vi "CRYGet Scale in Curves.vi"(11 "Graph VI Ref":refnum<vi>) -> (0 "Y min":dbl, 1 "Y max":dbl, 2 "X min":dbl, 3 "X max":dbl)   [LabVIEW 2013]
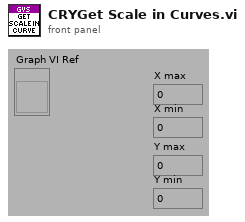
[diagram p1: front panel]
types:
  T1 = typedef "CRYData Cluster.ctl" = cluster{"Name":string, "Curve":cluster{"x":dbl, "y":dbl, "z":dbl}[], "X data":u16, "Y data":u16, "Z data":u16, "X axis":u16, "Y axis":u16, "Z axis":u16, "X unit":string, "Y unit":string, "Z unit":string, "X dB ref":dbl, "Y dB ref":dbl, "Z dB ref":dbl, "single val":bool, "protected":bool, "display X":bool, "display Y":bool, "display Z":bool, "Test Info":string, "Step No.":i32, "Plot Settings":cluster{"Color":u32, "Interpolation":u8, "Point Style":u8, "Line Style":u8, "Point Color":u32, "Line Width":u8, "Bar Plot Style":u8, "Fill To":i16}, "AutoProtect":bool}
  T2 = typedef "CRYWaveform Cluster.ctl" = cluster{"Waveform":cluster{"X0":dbl, "dX":dbl, "Y":sgl[]}, "X data":u16, "Y data":u16, "Y axis":u16, "X unit":string, "Y unit":string, "Y dB ref":dbl, "display Y":bool, "display X":bool, "Overload?":bool, "Test Info":string, "Step No.":i32, "Name":string, "protected":bool, "Sqc history":string[], "Signal Channel ID":i32, "Plot Settings":cluster{"Color":u32, "Interpolation":u8, "Point Style":u8, "Line Style":u8, "Point Color":u32, "Line Width":u8, "Bar Plot Style":u8, "Fill To":i16}, "AutoProtect":bool}
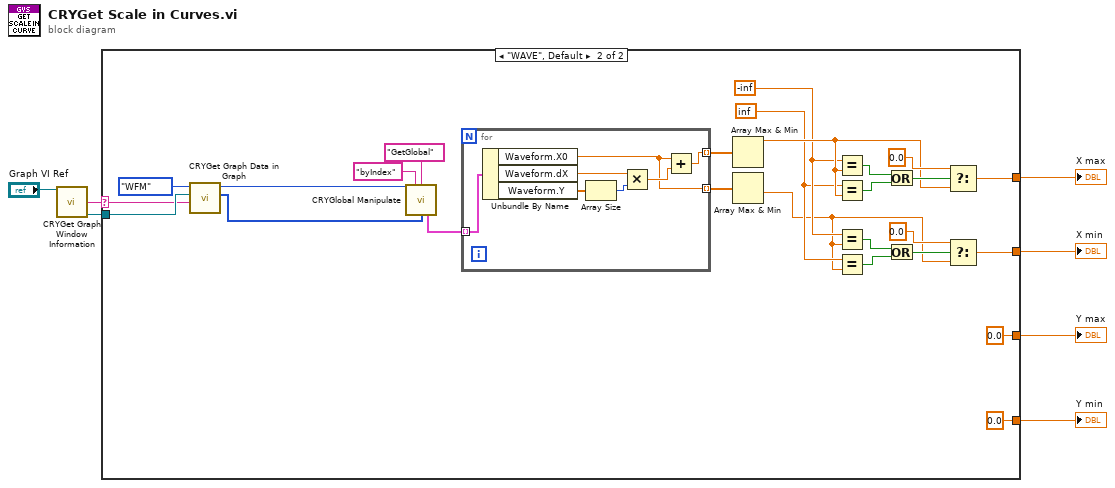
[diagram p0: block diagram]
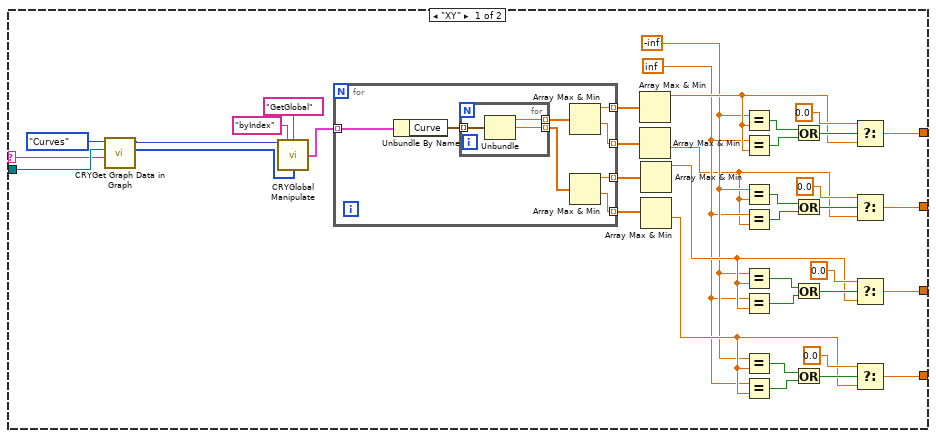
[diagram p2: hidden frame]
diagram:
  n1 = call "CRYGet Graph Window Information.vi"("pGraph VI In"="Graph VI Ref") -> ("Graph Type Out"=w2:string, "Legend Ref Out"=w1:refnum<vi>)  [unwired: 4 in, 9 out]
  n2 = case shown="\"WAVE\", Default" w2 {
    selector: w2 -> [w13 w64]
    tunnel: [w36 w75] -> w7
    tunnel: [w31 w70] -> w6
    tunnel: [w26 0.0 ("max value")] -> w5
    tunnel: [w21 0.0 ("max value")] -> w4
    tunnel: w1 -> [w14 w65]
    frame "XY" {
      w18 = -inf
      w17 = inf
      n3 = call "CRYGet Graph Data in Graph.vi"("Graph Type"=w13, "Legend Refnum"=w14, "Type In"=enum16{"Curves", "Values", "Results", "WFM"}."Curves") -> ("Rows"=w8:i32[], "Type Out"=w9:enum16{"Curves", "Values", "Results", "WFM"})  [unwired: 4 in, 3 out]
      n4 = call "CRYGlobal Manipulate.vi"("Type"=w9, "sOption"="byIndex", "sAction"="GetGlobal", "nData"=w8) -> ("Curves Out"=w11:T1[])  [unwired: 5 in, 6 out]
      n5 = for {
        tunnel: [w50] -> w42 mode=indexing
        tunnel: [w49] -> w43 mode=indexing
        tunnel: [w48] -> w44 mode=indexing
        tunnel: [w47] -> w45 mode=indexing
        tunnel: w11 -> [w46] mode=indexing
        n6 = Unbundle By Name(w46) -> ("Curve"=w53:cluster{"x":dbl, "y":dbl, "z":dbl}[])
        n7 = for {
          tunnel: w53 -> [w56] mode=indexing
          tunnel: [w55] -> w52 mode=indexing
          tunnel: [w54] -> w51 mode=indexing
          n8 = Unbundle(w56) -> ("x"=w55:dbl, "y"=w54:dbl)  [unwired: 1 out]
        }
        n9 = Array Max & Min(array=w52) -> (max value=w50:dbl, min value=w48:dbl)  [unwired: 2 out]
        n10 = Array Max & Min(array=w51) -> (max value=w49:dbl, min value=w47:dbl)  [unwired: 2 out]
      }
      n11 = Array Max & Min(array=w42) -> (max value=w37:dbl)  [unwired: 3 out]
      n12 = Array Max & Min(array=w44) -> (min value=w16:dbl)  [unwired: 3 out]
      n13 = Array Max & Min(array=w43) -> (max value=w19:dbl)  [unwired: 3 out]
      n14 = Array Max & Min(array=w45) -> (min value=w20:dbl)  [unwired: 3 out]
      n15 = Equal?(x=w18, y=w37) -> (x = y?=w41:bool)
      n16 = Equal?(x=w17, y=w37) -> (x = y?=w40:bool)
      n17 = Equal?(x=w18, y=w16) -> (x = y?=w32:bool)
      n18 = Equal?(x=w17, y=w16) -> (x = y?=w33:bool)
      n19 = Equal?(x=w18, y=w19) -> (x = y?=w30:bool)
      n20 = Equal?(x=w17, y=w19) -> (x = y?=w29:bool)
      n21 = Equal?(x=w18, y=w20) -> (x = y?=w22:bool)
      n22 = Equal?(x=w17, y=w20) -> (x = y?=w23:bool)
      n23 = Or(x=w41, y=w40) -> (x .or. y?=w39:bool)
      n24 = Or(x=w32, y=w33) -> (x .or. y?=w34:bool)
      n25 = Or(x=w30, y=w29) -> (x .or. y?=w28:bool)
      n26 = Or(x=w22, y=w23) -> (x .or. y?=w24:bool)
      n27 = Select(t=0.0 ("max value"), s=w39, f=w37) -> (s? t:f=w36:dbl)
      n28 = Select(t=0.0 ("max value"), s=w34, f=w16) -> (s? t:f=w31:dbl)
      n29 = Select(t=0.0 ("max value"), s=w28, f=w19) -> (s? t:f=w26:dbl)
      n30 = Select(t=0.0 ("max value"), s=w24, f=w20) -> (s? t:f=w21:dbl)
    }
    frame "WAVE", Default {
      w69 = -inf
      w68 = inf
      n31 = call "CRYGet Graph Data in Graph.vi"("Graph Type"=w64, "Legend Refnum"=w65, "Type In"=enum16{"Curves", "Values", "Results", "WFM"}."WFM") -> ("Rows"=w58:i32[], "Type Out"=w57:enum16{"Curves", "Values", "Results", "WFM"})  [unwired: 4 in, 3 out]
      n32 = call "CRYGlobal Manipulate.vi"("Type"=w57, "sOption"="byIndex", "sAction"="GetGlobal", "nData"=w58) -> ("WFM Out"=w61:T2[])  [unwired: 5 in, 6 out]
      n33 = for {
        tunnel: [w85] -> w81 mode=indexing
        tunnel: [w84] -> w82 mode=indexing
        tunnel: w61 -> [w83] mode=indexing
        n34 = Unbundle By Name(w83) -> ("Waveform.X0"=w84:dbl, "Waveform.dX"=w88:dbl, "Waveform.Y"=w89:sgl[])
        n35 = Array Size(array=w89) -> (size(s)=w87:i32)
        n36 = Multiply(x=w88, y=w87) -> (x*y=w86:dbl)
        n37 = Add(x=w84, y=w86) -> (x+y=w85:dbl)
      }
      n38 = Array Max & Min(array=w81) -> (max value=w76:dbl)  [unwired: 3 out]
      n39 = Array Max & Min(array=w82) -> (min value=w67:dbl)  [unwired: 3 out]
      n40 = Equal?(x=w69, y=w76) -> (x = y?=w80:bool)
      n41 = Equal?(x=w68, y=w76) -> (x = y?=w79:bool)
      n42 = Equal?(x=w69, y=w67) -> (x = y?=w71:bool)
      n43 = Equal?(x=w68, y=w67) -> (x = y?=w72:bool)
      n44 = Or(x=w80, y=w79) -> (x .or. y?=w78:bool)
      n45 = Or(x=w71, y=w72) -> (x .or. y?=w73:bool)
      n46 = Select(t=0.0 ("max value"), s=w78, f=w76) -> (s? t:f=w75:dbl)
      n47 = Select(t=0.0 ("max value"), s=w73, f=w67) -> (s? t:f=w70:dbl)
    }
  }
  "X max" <- w7
  "X min" <- w6
  "Y max" <- w5
  "Y min" <- w4
